vi "FoodPlacing.vi"(8 "error in (no error)":errorcluster, 11 "Snake in":refnum<class "Snake.lvclass">) -> (0 "error out":errorcluster, 3 "Snake out":refnum<class "Snake.lvclass">)   [LabVIEW 2014, in "Snake.lvclass"]
uses:
  Snake.lvclass
  Snake.lvclass/Snake.ctl
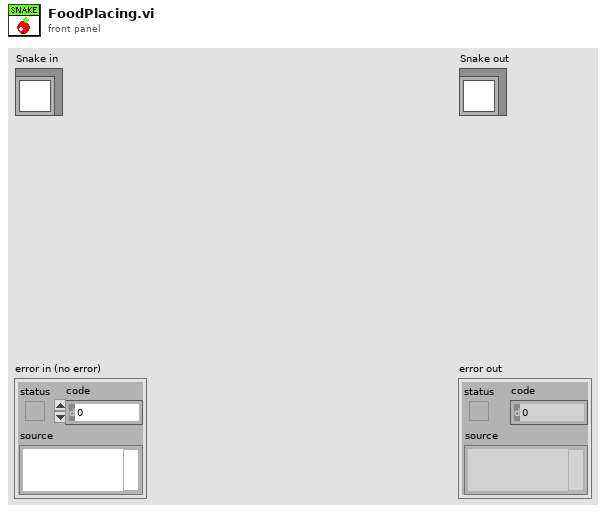
[diagram p1: front panel]
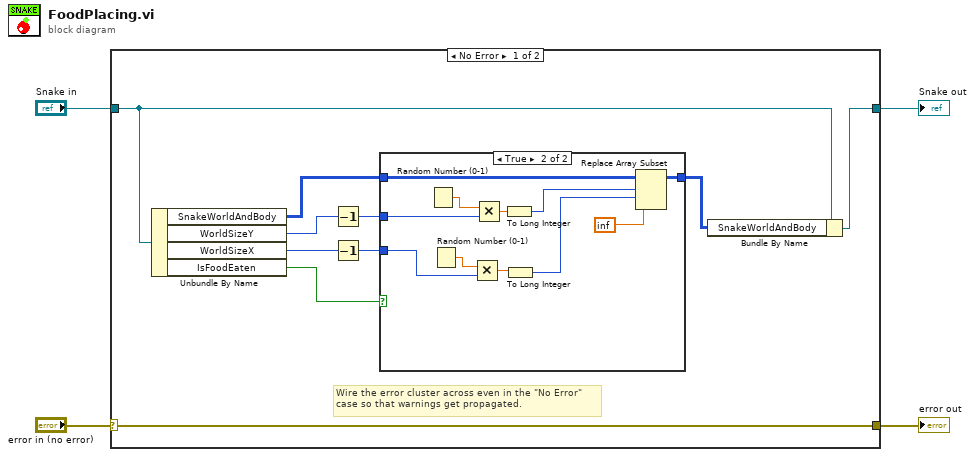
[diagram p0: block diagram]
diagram:
  n1 = case shown="No Error" "error in (no error)" {
    selector: "error in (no error)" -> [w14 w28]
    tunnel: [w14 w28] -> w3
    tunnel: [w13 w27] -> w1
    tunnel: "Snake in" -> [w12 w27]
    frame No Error {
      # "Wire the error cluster across even in the \"No Error\"\ncase so that warnings get propagated."
      n2 = Unbundle By Name(w12) -> ("SnakeWorldAndBody"=w8:u32[][], "WorldSizeY"=w10:i32, "WorldSizeX"=w9:i32, "IsFoodEaten"=w11:bool)
      n3 = Decrement(x=w10) -> (x-1=w6:i32)
      n4 = Decrement(x=w9) -> (x-1=w5:i32)
      n5 = case shown="True" w11 {
        tunnel: w6 -> [_ w19]
        tunnel: w5 -> [_ w18]
        tunnel: w8 -> [w15 w17]
        tunnel: [w15 w16] -> w7
        frame False {
        }
        frame True {
          n6 = Random Number (0-1)() -> (number: 0 to 1=w25:dbl)
          n7 = Random Number (0-1)() -> (number: 0 to 1=w26:dbl)
          n8 = Multiply(x=w26, y=w18) -> (x*y=w24:dbl)
          n9 = Multiply(x=w25, y=w19) -> (x*y=w23:dbl)
          n10 = To Long Integer(number=w23) -> (32bit integer=w21:i32)
          n11 = To Long Integer(number=w24) -> (32bit integer=w22:i32)
          n12 = Replace Array Subset(array=w17, new element=inf, index (row)=w21, index (col)=w22) -> (w16:u32[][])
        }
      }
      n13 = Bundle By Name(cluster=w12, "SnakeWorldAndBody"=w7) -> (w13:refnum<class "Snake.lvclass">)
    }
    frame Error {
    }
  }
  "error out" <- w3
  "Snake out" <- w1
